vi "GUI_Plasma2SuperGUI_capillaries.vi"() -> ()   [LabVIEW 2013]
uses:
  Shared/GUI_Template/GUI_master/tcp_new_data_event.ctl
  Shared/GUI_Template/GUI_master/tcp new data cluster.ctl
  Device Drivers/DG645/subVIs/TriggerSource_TypDef.ctl
panel:
  out "reading.var 1::12":dbl=25.5 caption="Cap Temp" min=0.0 max=400.0 format="%_4f"
  in  "GUIdevice 12":string="P2-PR4000"
  in  "Amplitude.Ch EF::2":dbl=0.001 caption="Trigger Rate [Hz]" min=0.5 max=5.0 format="%_2f"
  in  "Polarity.Ch EF::2":string caption="polarity EF"
  in  "laser":bool
  in  "ignore pressure interlock":bool
  in  "Reading.Channel 1::7":dbl=0.001 caption="OUT (J)" min=0.0 max=0.0 format="%_3p"
  in  "Reading.Channel 2::7":dbl=0.001 caption="IN (J)" min=0.0 max=0.0 format="%_3p"
  in  "correction":dbl=1.0 caption="Trans multiplier" min=0.0 max=0.0 format="%_3p"
  out "Transmission":dbl=0.001 caption="%" min=0.0 max=0.0 format="%_3p"
  out "Output E":dbl=0.001 caption="OUT (J)" min=0.0 max=0.0 format="%_3p"
  out "Input E":dbl=0.001 caption="IN (J)" min=0.0 max=0.0 format="%_3p"
  in  "Delay.Ch E::2":dbl=25.5 caption="Q-switch" min=-1.0 max=2.0 format="%_4p"
  in  "GUIdevice 7":string="P2-HeatEnergy"
  in  "position::6":dbl=25.5 caption="Mode imager stage location" min=0.0 max=400.0 format="%_4f"
  in  "uangle::3":dbl=0.001 caption="u angle [deg]" min=-6.0 max=6.0 format="%_4p"
  in  "vangle::3":dbl=0.001 caption="v angle [deg]" min=-2.0 max=2.0 format="%_4p"
  in  "wangle::3":dbl=0.001 caption="w angle [deg]" min=-2.0 max=2.0 format="%_4p"
  in  "ypos::3":dbl=0.001 caption="hex y [mm]" min=-25.0 max=25.0 format="%_4p"
  in  "zpos::3":dbl=0.001 caption="hex z [mm]" min=-12.0 max=12.0 format="%_4p"
  in  "xpos::3":dbl=0.001 caption="hex x [mm]" min=-20.0 max=20.0 format="%_4p"
  in  "GUIdevice 6":string="P2-ImagingStage"
  out "bar pressure 2":dbl=25.5 caption="Baratron 2 (torr)" min=-10.0 max=10.0 format="%_4f"
  out "bar pressure":dbl=25.5 caption="Baratron 1 (torr)" min=-10.0 max=10.0 format="%_4f"
  out "flow::11":dbl=25.5 caption="PR4000 Flow" min=0.0 max=0.0 format="%_4f"
  in  "valve::11":bool caption="Valve"
  in  "pressure::11":dbl=25.5 caption="PR4000 Pressure" min=0.0 max=500.0 format="%_4f"
  in  "AI_mean.Channel 1::9":dbl=25.5 caption="Baratron 2 (V)" min=-10.0 max=10.0 format="%_4f"
  in  "GUIdevice 5":string="P2-hexapod"
  in  "voltage::4":dbl=25.5 caption="Discharge HV" min=-9999999.0 max=9999999.0 format="%_4f"
  in  "Trigger Control":enum32{"Trigger", "Single Shot"}(tab)
  in  "Trigger.Rate::2":dbl=0.001 caption="Trigger Rate [Hz]" min=0.001 max=1000.0 format="%_2f"
  in  "fire::2":string caption="Fire Status"
  in  "Fire":bool
  in  "continuous ms wait":u32=1000
  in  "continuous":bool
  in  "Trigger.Source::2":T1 caption="Trigger Source"
  in  "GUIdevice 4":string="P2-capHV"
  in  "GUIdevice 3":string="P2-hexapod"
  in  "GUIdevice 2":string="P2-SRS"
  out "pressure chart 2":dbl(graph) caption="PR4000 pressure"
  in  "AI_mean.Channel 0::9":dbl=25.5 caption="Baratron V" min=-10.0 max=10.0 format="%_4f"
  out "pressure chart":dbl(graph) caption="Baratron pressure"
  in  "GUIdevice 11":string="P2-PR4000"
  in  "GUIdevice 9":string="P2-DAQ6210"
  out "error IO 2":errorcluster
  in  "insert tag":bool=TRUE
  out "tcp data event":T2
  in  "stop":bool
  in  "UDP error message":string
  # "Plasma 2 Capillary GUI"
  # "Heater energy"
  # "Hexapod Control"
  # "Pressures"
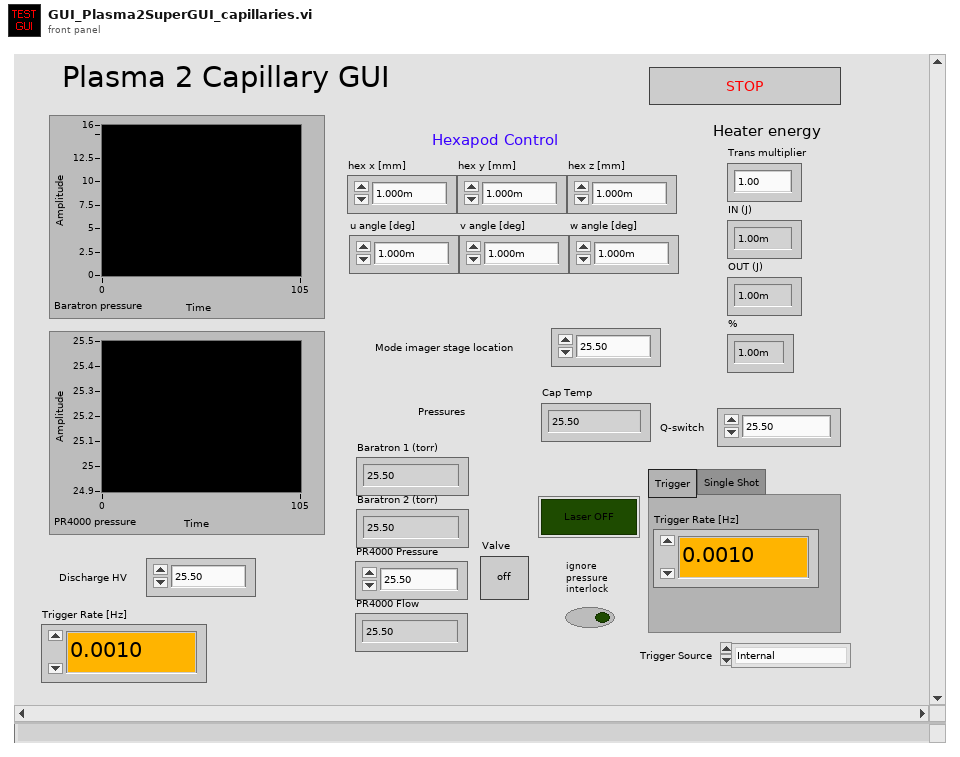
[diagram p1: front panel]
types:
  T1 = typedef "TriggerSource_TypDef.ctl" = enum16{"Internal", "External rising edges", "External falling edges", "Single shot external rising edges", "Single shot external falling edges", "Single shot", "Line"}
  T2 = typedef "tcp_new_data_event.ctl" = refnum<user-event>
  T3 = typedef "tcp new data cluster.ctl" = cluster{"EventEnum":enum16{"new data", "connection status update"}, "Device name":string}
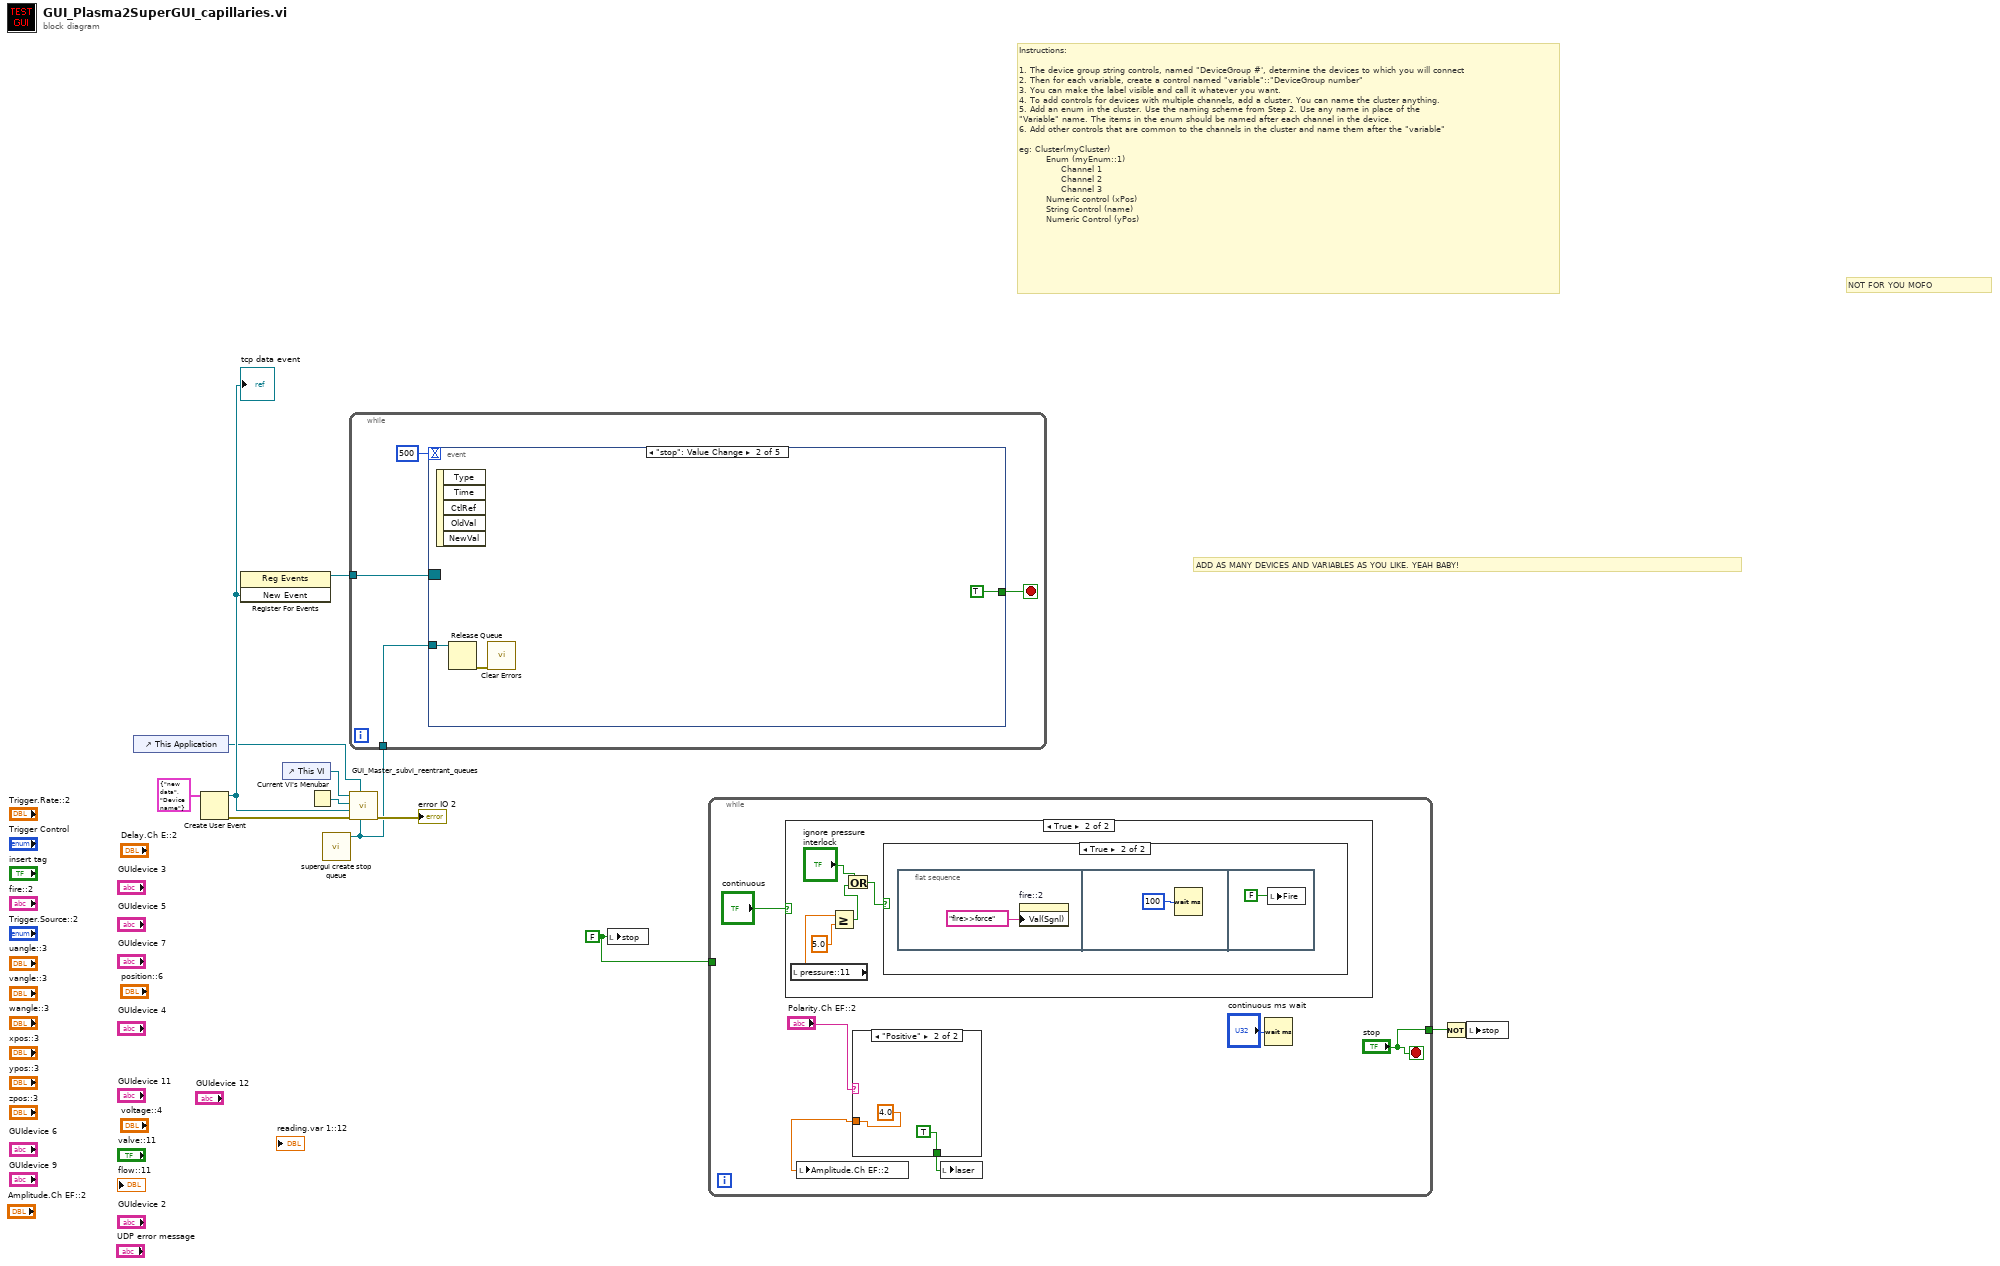
[diagram p0: block diagram]
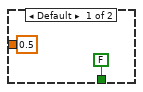
[diagram p2: hidden frame]
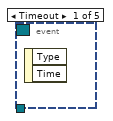
[diagram p5: hidden frame]
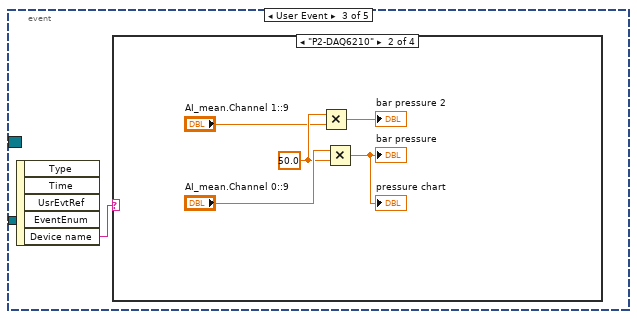
[diagram p6: hidden frame]
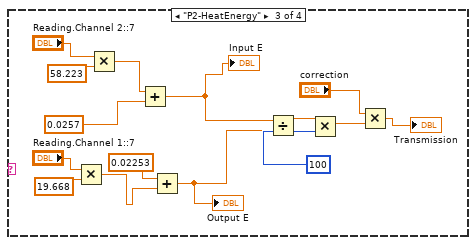
[diagram p8: hidden frame]
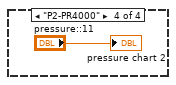
[diagram p9: hidden frame]
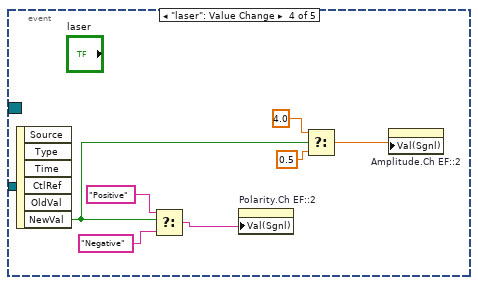
[diagram p10: hidden frame]
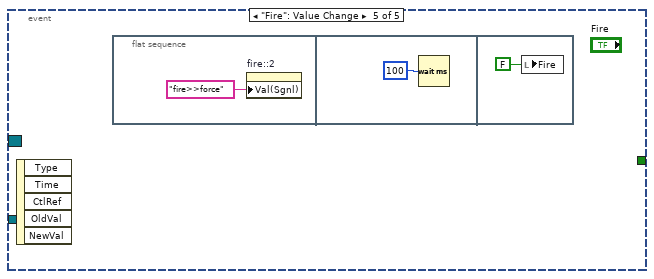
[diagram p11: hidden frame]
diagram:
  w2 = FALSE ("stop")
  # "Instructions:\n\n1. The device group string controls, named \"DeviceGroup #', determine the devices to which you will connect\n2. Then for each variable, create a control named \"variable\"::\"DeviceGroup number\"\n3. You can make the label visible and call it whatever you want.\n4. To add controls for devices with multiple channels, add a cluster. You can name the cluster anything.\n5. Add an enum in the cluster. Use the naming scheme from Step 2. Use any name in place of the \n\"Variable\" name. The items in the enum should be named after each channel in the device. \n6. Add other controls that are common to the channels in the cluster and name them after the \"variable\"\n\neg: Cluster(myCluster)\n         Enum (myEnum::1)\n              Channel 1 \n              Channel 2\n              Channel 3\n         Numeric control (xPos)\n         String Control (name)\n         Numeric Control (yPos)"
  # "ADD AS MANY DEVICES AND VARIABLES AS YOU LIKE. YEAH BABY!"
  # "NOT FOR YOU MOFO"
  n1 = control-ref of="This Application"() -> (w5:refnum<vi>)
  n2 = Create User Event(user event datatype=T3 {"EventEnum"=enum."new data", "Device name"="Device name"} ("New Event")) -> (user event=w7:refnum<user-event>, error out=w12:errorcluster)  [unwired: 1 in]
  "tcp data event" <- w7
  n3 = register-events(w7) -> (reference out=w6:refnum<event-registration>)  [unwired: 2 in, 1 out]
  n4 = control-ref of="This VI"() -> (w9:refnum<vi>)
  n5 = Current VI's Menubar() -> (w10:refnum<k9>)
  n6 = call "supergui create stop queue.vi"() -> ("STOP Queue out"=w1:refnum<queue>)  [unwired: 11 in]
  n7 = while {
    tunnel: w6 -> [w16]
    tunnel: w1 -> [w13]
    stop <- w14 stop-if-true
    n8 = event shown="[1] \"stop\": Value Change" {
      selector: w16 -> [_ _ _ _ _]
      dyn-events: _ -> [_ _ _ _ _]
      timeout: 500 -> [_ _ _ _ _]
      tunnel: [_ TRUE _ _ _] -> w14
      tunnel: w13 -> [_ w18 _ _ _]
      event Timeout {
        n9 = event-data() -> ()  [unwired: 1 in, 2 out]
      }
      event "stop": Value Change {
        n10 = event-data() -> ()  [unwired: 1 in, 5 out]
        n11 = Release Queue(queue=w18) -> (error out=w17:errorcluster)  [unwired: 2 in, 2 out]
        n12 = call <vilib>:"Clear Errors.vi"("error in (no error)"=w17) -> ()  [unwired: 6 in, 1 out]
      }
      event User Event {
        n13 = event-data() -> ("Device name"=w20:string)  [unwired: 1 in, 4 out]
        n14 = case shown="\"P2-DAQ6210\"" w20 {
          frame Default {
          }
          frame "P2-DAQ6210" {
            w23 = 50.0 ("y")
            n15 = Multiply(x=w23, y="AI_mean.Channel 1::9") -> (x*y=→"bar pressure 2":dbl)
            n16 = Multiply(x="AI_mean.Channel 0::9", y=w23) -> (x*y=→"pressure chart" →"bar pressure":dbl)
          }
          frame "P2-HeatEnergy" {
            n17 = Multiply(x="Reading.Channel 1::7", y=19.668) -> (x*y=w26:dbl)
            n18 = Multiply(x="Reading.Channel 2::7", y=58.223) -> (x*y=w31:dbl)
            n19 = Add(x=w31, y=0.0257) -> (x+y=w27:dbl)
            "Input E" <- w27
            n20 = Add(x=0.02253, y=w26) -> (x+y=w32:dbl)
            "Output E" <- w32
            n21 = Divide(x=w27, y=w32) -> (x/y=w39:dbl)
            n22 = Multiply(x=w39, y=100) -> (x*y=w37:dbl)
            n23 = Multiply(x="correction", y=w37) -> (x*y=→"Transmission":dbl)
          }
          frame "P2-PR4000" {
            "pressure chart 2" <- "pressure::11"
          }
        }
      }
      event "laser": Value Change {
        n24 = event-data() -> ("NewVal"=w45:bool)  [unwired: 1 in, 5 out]
        n25 = Select(t="Positive" ("Polarity.Ch EF::2"), s=w45, f="Negative" ("Polarity.Ch EF::2")) -> (s? t:f=w46:string)
        n26 = property on="Polarity.Ch EF::2" class="Str"("Val(Sgnl)"=w46) -> ()  [unwired: 2 in, 2 out]
        n27 = Select(t=4.0 ("Amplitude.Ch EF::2"), s=w45, f=0.5 ("Amplitude.Ch EF::2")) -> (s? t:f=w42:dbl)
        n28 = property on="Amplitude.Ch EF::2" class="DigNum (strict)"("Val(Sgnl)"=w42) -> ()  [unwired: 2 in, 2 out]
      }
      event "Fire": Value Change {
        n29 = event-data() -> ()  [unwired: 1 in, 5 out]
        n30 = flat-sequence {
          frame #0 {
            n31 = property on="fire::2" class="Str"("Val(Sgnl)"="fire>>force" ("Value (Signaling)")) -> ()  [unwired: 2 in, 2 out]
          }
          frame #1 {
            n32 = Wait (ms)(milliseconds to wait=u32 100) -> ()  [unwired: 1 out]
          }
          frame #2 {
            n33 = local write "Fire"(FALSE ("Fire")) -> ()
          }
        }
      }
    }
  }
  n34 = call "GUI_Master_subvi_reentrant_queues.vi"("STOP Queue in"=w1, "This Application"=w5, "error in (no error)"=w12, "tcp data event"=w7, "Caller menu reference"=w10, "Caller VI ref"=w9) -> ("error out"=→"error IO 2":errorcluster)  [unwired: 5 in]
  n35 = local write "stop"(w2) -> ()
  n36 = while {
    tunnel: ["stop"] -> w4
    tunnel: w2 -> [_]
    stop <- "stop" stop-if-true
    n37 = case shown="True" "continuous" {
      frame False {
      }
      frame True {
        n38 = local read "pressure::11"() -> (w66:dbl)
        n39 = Greater Or Equal?(x=w66, y=5.0) -> (x >= y?=w63:bool)
        n40 = Or(x="ignore pressure interlock", y=w63) -> (x .or. y?=w62:bool)
        n41 = case shown="True" w62 {
          frame False {
          }
          frame True {
            n42 = flat-sequence {
              frame #0 {
                n43 = property on="fire::2" class="Str"("Val(Sgnl)"="fire>>force" ("Value (Signaling)")) -> ()  [unwired: 2 in, 2 out]
              }
              frame #1 {
                n44 = Wait (ms)(milliseconds to wait=u32 100) -> ()  [unwired: 1 out]
              }
              frame #2 {
                n45 = local write "Fire"(FALSE ("Fire")) -> ()
              }
            }
          }
        }
      }
    }
    n46 = case shown="\"Positive\"" "Polarity.Ch EF::2" {
      tunnel: [FALSE ("laser") TRUE ("laser")] -> w53
      tunnel: [0.5 ("Amplitude.Ch EF::2") 4.0 ("Amplitude.Ch EF::2")] -> w54
      frame Default {
      }
      frame "Positive" {
      }
    }
    n47 = local write "Amplitude.Ch EF::2"(w54) -> ()
    n48 = local write "laser"(w53) -> ()
    n49 = Wait (ms)(milliseconds to wait="continuous ms wait") -> ()  [unwired: 1 out]
  }
  n50 = Not(x=w4) -> (.not. x?=w3:bool)
  n51 = local write "stop"(w3) -> ()
